vi "GetInstance.vi"(5 "error in (no error)":errorcluster) -> (14 "reference out":refnum<class "UmlEditor.lvclass">, 16 "DVRRefOut":refnum<data-value>, 19 "error out":errorcluster)   [LabVIEW 2016, in "UmlEditor.lvclass"]
uses:
  <resource>/Framework/Providers/Open_GDS/UML/UmlEditor_class/UmlEditor.lvclass
  <resource>/Framework/Providers/Open_GDS/UML/UmlEditor_class/protected/ObjectAttributes.ctl
  <resource>/Framework/Providers/Open_GDS/UML/UmlEditor_class/EventData.ctl
  <resource>/Framework/Providers/Open_GDS/UML/UMLEditor/UMLEditor_SyncOptions.ctl
  <resource>/Framework/Providers/Open_GDS/UML/UmlEditor_class/IniParamsType.ctl
panel:
  in  "DummyRef(hidden)":refnum<class "UmlEditor.lvclass">
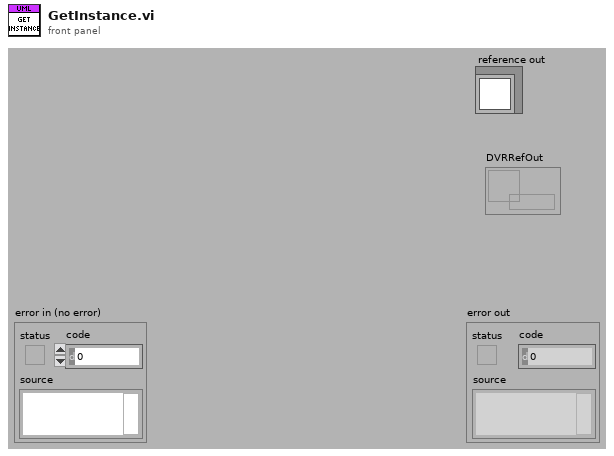
[diagram p1: front panel]
types:
  T1 = enum16{"Create or look up existing", "Look up existing"}
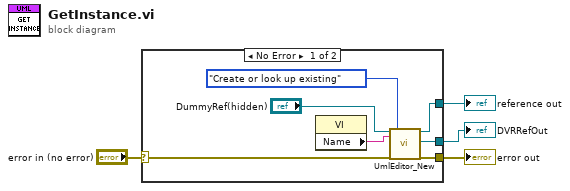
[diagram p0: block diagram]
diagram:
  n1 = case shown="No Error" "error in (no error)" {
    selector: "error in (no error)" -> [w11 w12]
    tunnel: [w10 w12] -> w4
    tunnel: [w9 _] -> w2
    tunnel: [w5 _] -> w1
    frame No Error {
      n2 = property class="VI"() -> ("Name"=w6:string)  [unwired: 2 in, 2 out]
      n3 = call <resource>:"UmlEditor_New.vi"("reference in"="DummyRef(hidden)", "Object name"=w6, "error in (no error)"=w11, "CreateMethod(Create or look up existing)"=T1."Create or look up existing" ("Create method")) -> ("reference out"=w9:refnum<class "UmlEditor.lvclass">, "DVRRefOut"=w5:refnum<data-value>, "error out"=w10:errorcluster)  [unwired: 3 in, 10 out]
    }
    frame Error {
    }
  }
  "error out" <- w4
  "reference out" <- w2
  "DVRRefOut" <- w1
